vi "FFT_part2.vi"() -> ()   [LabVIEW 2020]
uses:
  <vilib>/Analysis/2dsp.llb/Real FFT.vi
  <vilib>/Waveform/WDTOps.llb/WDT Get Waveform Time Array DBL.vi
  <vilib>/Waveform/WDTOps.llb/WDT Get Final Time Value DBL.vi
  <vilib>/express/express analysis/Spectral/Block/exnSpectralBlock spectral measurements power poly.vi
  <vilib>/express/express analysis/Spectral/Block/exnSpectralBlock spectral measurements power WFM.vi
  <vilib>/express/express analysis/Spectral/Block/exnSpectralBlock spectral measurements power DDT.vi
  <vilib>/express/express analysis/Spectral/XNode/ExpressSpectralMeasurementsBlockNode.xnode
  <vilib>/Analysis/NI_AALPro.lvlib
panel:
  out "Manual Amplitude Spectrum":cluster{"X":dbl, "Y":dbl}[](graph)
  out "Manual Power Spectrum (normalised but no complex no.s)":cluster{"X":dbl, "Y":dbl}[](graph)
  in  "Power Spectrum Reconstruction":T1(tab)
  out "Power Spectrum Array":cdb[](array[numeric])
  out "Frequency Array":dbl[](array[numeric])
  out "FFT init Array":dbl[](array[numeric])
  out "FFT array":dbl[](array[numeric])
  out "FFT Array":cdb[](array[numeric])
  out "Frequency Array 2":dbl[](array[numeric])
  out "Graph From Arrays":cluster{"X":dbl, "Y":dbl}[](graph)
  out "element":dbl
  in  "WaveForm DataSets":T2(tab)
  out "Start Time":timestamp
  out "Sampling Time Interval":dbl
  out "Data Array":dbl[](array[numeric])
  out "Sampling Frequency":dbl
  out "Final Time of WaveForm":timestamp
  out "Time Array":timestamp[](array[timestamp])
  out "Array index indicator (time domain)":waveform(dbl)
  out "initialized array":dbl[](array[numeric])
  out "Array of Indices":dbl[](array[numeric])
  out "Array of Time":dbl[](array[numeric])
  out "Data vs Time Array":dbl[][](array[numeric])
  out "Data vs Time array (Transposed)":dbl[][](array[numeric])
  out "Array after indexing":dbl[](array[numeric])
  out "size of wav":i32
  in  "index":i32
  out "FFT array size indicator":i32
  out "Filtered Spectral Measurement":dynamicdata(graph)
  out "Spectral Measurement":cluster{"f0":dbl, "df":dbl, "magnitude":dbl[]}(graph)
  in  "shift?":bool
  in  "Array size control":i32=-1
  out "Fast Fourier Transform Graph":dbl[](graph)
  out "Amplitude vs Time (Chart)":waveform(dbl)(graph)
  out "Amplitude vs Time (Graph)":waveform(dbl)(graph)
  in  "path":path
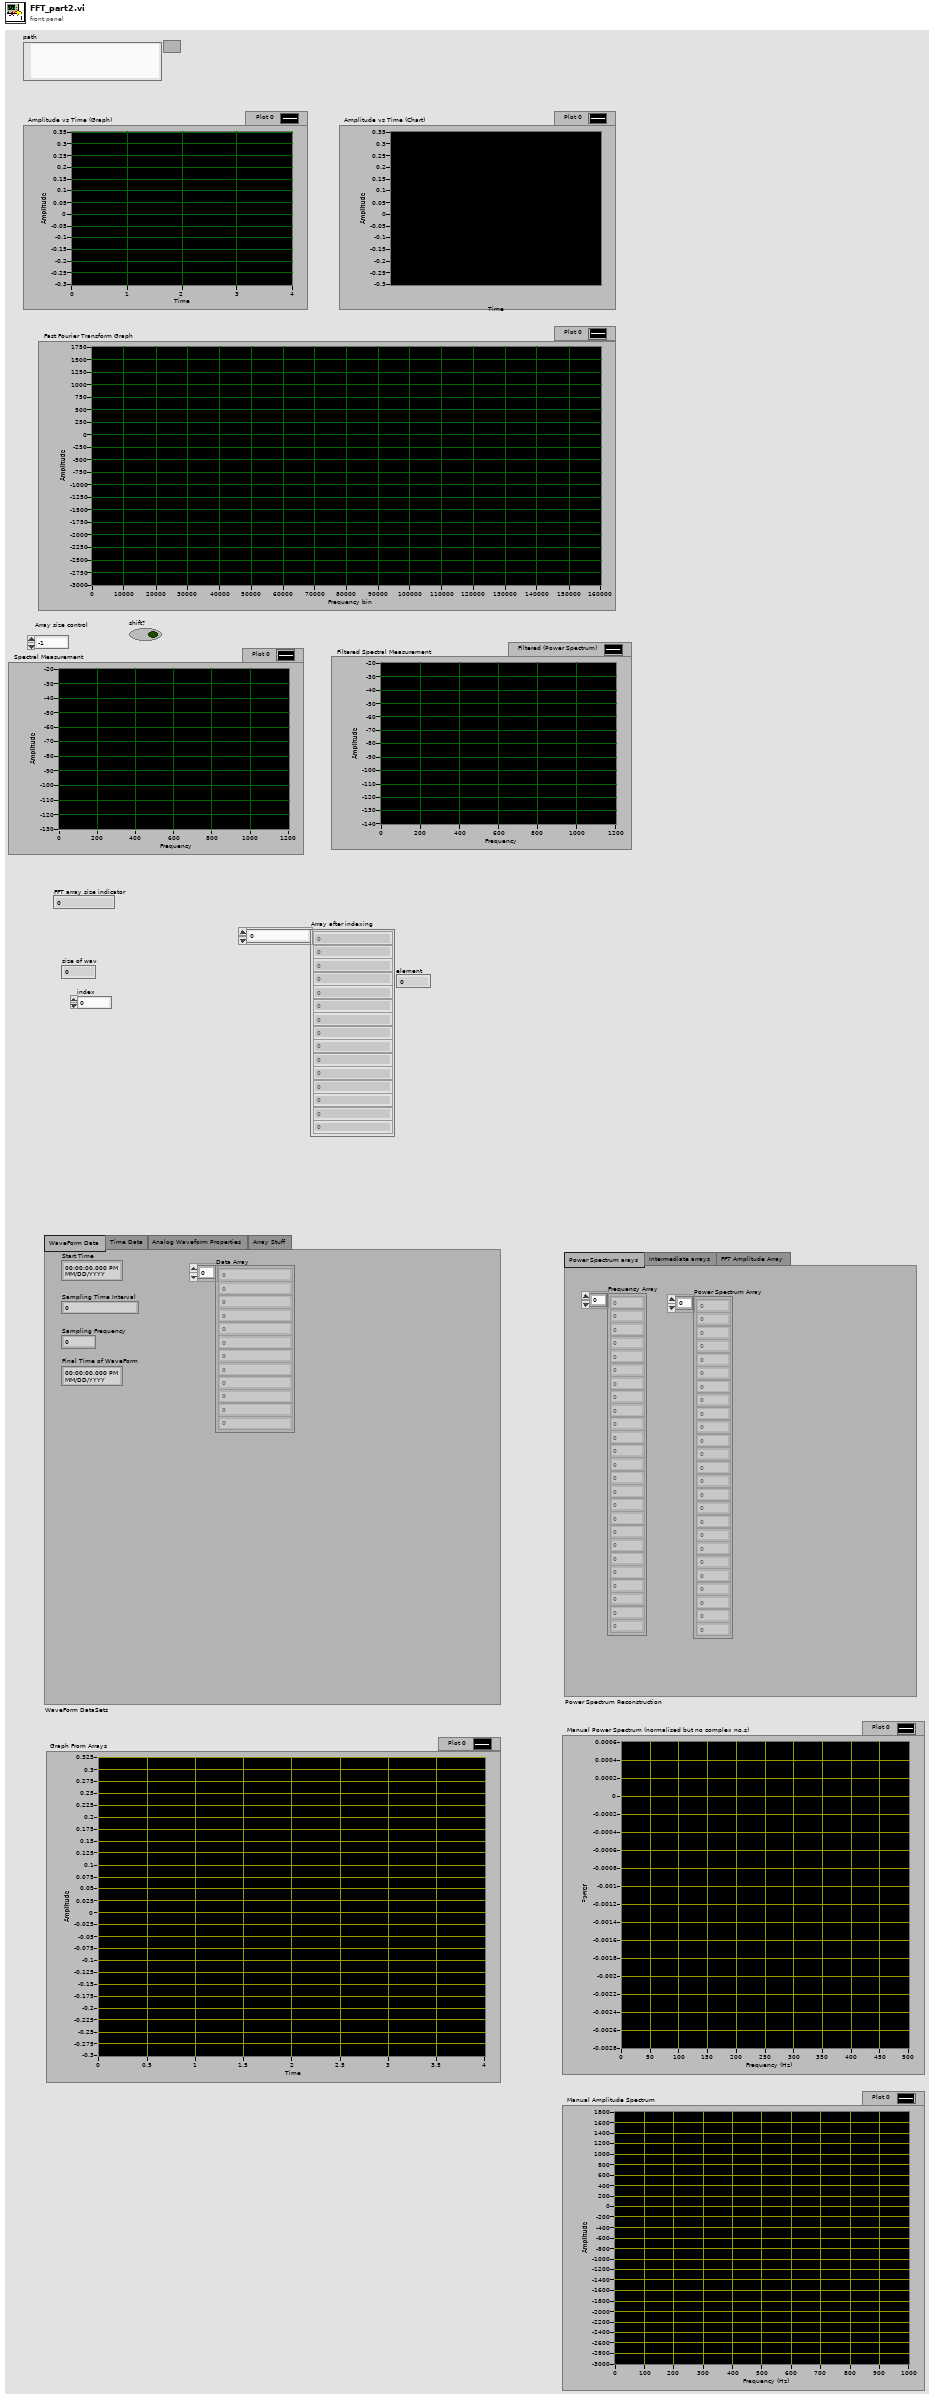
[diagram p1: front panel]
types:
  T1 = enum32{"Power Spectrum arays", "Intermediate arrays", "FFT Amplitude Array"}
  T2 = enum32{"WaveForm Data", "Time Data", "Analog Waveform Properties", "Array Stuff"}
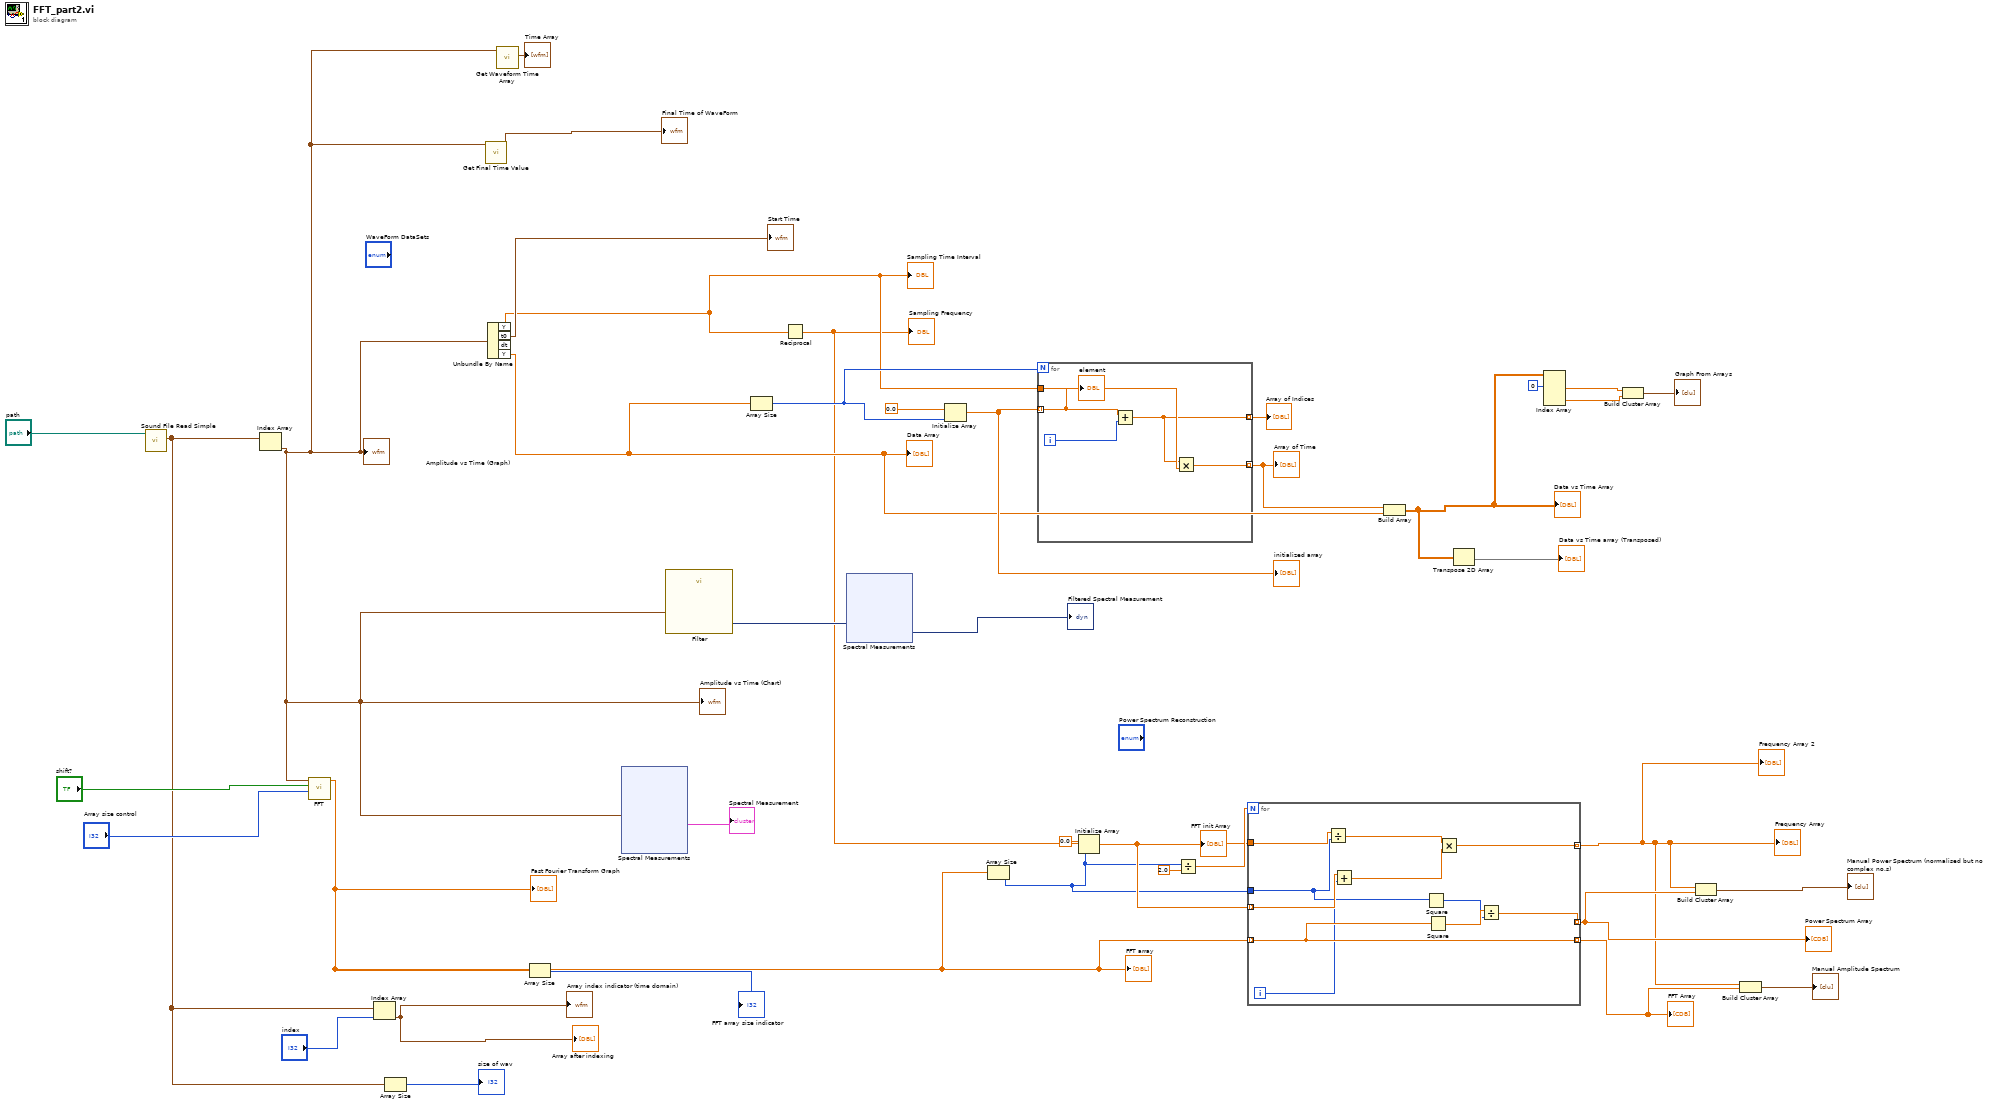
[diagram p0: block diagram]
diagram:
  n1 = call <vilib>:"Sound File Read Simple.vi"("path"="path") -> ("data"=w30:waveform(dbl)[])  [unwired: 7 in, 3 out]
  n2 = Index Array(array=w30) -> (element=w27:waveform(dbl))  [unwired: 1 in]
  "Amplitude vs Time (Graph)" <- w27
  "Amplitude vs Time (Chart)" <- w27
  n3 = call-poly <vilib>:"FFT.vi"("FFT size"="Array size control", "shift?"="shift?", "X"=w27) -> ("FFT {X}"=w9:cdb[])  [unwired: 7 in, 1 out]
  "Fast Fourier Transform Graph" <- w9
  "FFT array" <- w9
  n4 = Index Array(array=w30, index="index") -> (element=→"Array index indicator (time domain)" →"Array after indexing":waveform(dbl))
  n5 = Array Size(array=w30) -> (size(s)=→"size of wav":i32)
  n6 = call-poly <vilib>:"Get Final Time Value.vi"("waveform in"=w27) -> ("tf"=→"Final Time of WaveForm":timestamp)  [unwired: 8 in, 2 out]
  n7 = Unbundle By Name(w27) -> ("t0"=→"Start Time":timestamp, "dt"=w22:dbl, "Y"=w19:dbl[])  [unwired: 1 out]
  "Sampling Time Interval" <- w22
  "Data Array" <- w19
  n8 = call-poly <vilib>:"Get Waveform Time Array.vi"("waveform in"=w27) -> ("X array"=→"Time Array":timestamp[])  [unwired: 9 in, 1 out]
  n9 = Array Size(array=w9) -> (size(s)=→"FFT array size indicator":i32)
  n10 = xnode "Spectral Measurements"("Signals"=w27) -> ("Power Spectrum"=→"Spectral Measurement":cluster{"f0":dbl, "df":dbl, "magnitude":dbl[]})  [unwired: 1 in, 1 out]
  n11 = call "Filter"("Signal"=w27) -> ("Filtered Signal"=w36:dynamicdata)  [unwired: 9 in, 1 out]
  n12 = Array Size(array=w19) -> (size(s)=w24:i32)
  n13 = Reciprocal(x=w22) -> (1/x=w6:dbl)
  "Sampling Frequency" <- w6
  n14 = xnode "Spectral Measurements"("Signals"=w36) -> ("Power Spectrum"=→"Filtered Spectral Measurement":dynamicdata)  [unwired: 1 in, 1 out]
  n15 = Initialize Array(0.0 ("element"), w24) -> (w21:dbl[])
  "initialized array" <- w21
  n16 = Array Size(array=w9) -> (size(s)=w7:i32)
  n17 = for {
    N: w24 -> [_]
    tunnel: w21 -> [w45] mode=indexing
    tunnel: [w42] -> w23 mode=indexing
    tunnel: w22 -> [w43]
    tunnel: [w41] -> w20 mode=indexing
    i -> [w44]
    n18 = Add(x=w45, y=w44) -> (x+y=w42:dbl)
    n19 = Multiply(x=w42, y=w43) -> (x*y=w41:dbl)
    "element" <- w45
  }
  "Array of Indices" <- w23
  "Array of Time" <- w20
  n20 = Initialize Array(0.0 ("element"), w7) -> (w8:dbl[])
  "FFT init Array" <- w8
  n21 = Divide(x=w7, y=2.0) -> (x/y=w10:dbl)
  n22 = for {
    N: w10 -> [_]
    tunnel: w9 -> [w56] mode=indexing
    tunnel: w8 -> [w55] mode=indexing
    tunnel: [w56] -> w2 mode=indexing
    tunnel: [w46] -> w5 mode=indexing
    tunnel: w7 -> [w49]
    tunnel: w6 -> [w52]
    tunnel: [w50] -> w3 mode=indexing
    i -> [w54]
    n23 = Divide(x=w52, y=w49) -> (x/y=w51:dbl)
    n24 = Add(x=w55, y=w54) -> (x+y=w53:dbl)
    n25 = Square(x=w49) -> (x^2=w47:i32)
    n26 = Square(x=w56) -> (x^2=w48:cdb)
    n27 = Multiply(x=w51, y=w53) -> (x*y=w50:dbl)
    n28 = Divide(x=w48, y=w47) -> (x/y=w46:cdb)
  }
  "FFT Array" <- w2
  "Power Spectrum Array" <- w5
  "Frequency Array" <- w3
  "Frequency Array 2" <- w3
  n29 = Build Array(w20, w19) -> (w17:dbl[][])
  "Data vs Time Array" <- w17
  n30 = Transpose 2D Array(2D array=w17) -> (transposed array=→"Data vs Time array (Transposed)":dbl[][])
  n31 = Index Array(array=w17, index (row) #1=0 ("index (row)")) -> (element #1=w15:dbl[], element #2=w14:dbl[])  [unwired: 3 in]
  n32 = Build Cluster Array(w15, w14) -> (→"Graph From Arrays":cluster{dbl, dbl}[])
  n33 = Build Cluster Array(w3, w5) -> (→"Manual Power Spectrum (normalised but no complex no.s)":cluster{dbl, cdb}[])
  n34 = Build Cluster Array(w3, w2) -> (→"Manual Amplitude Spectrum":cluster{dbl, cdb}[])
